vi "filter taps.vi"(8 "error in (no error)":errorcluster, 10 "filter parameters":T1={"Alpha"=0.5, "Filter Length"=6, "TX Filter"=enum."Root Raised Cos"} {"Alpha" format="%.2f"}, 11 "Samples Per Symbol (16)":i32=16) -> (2 "matched filter coefficients":dbl[](array[numeric]), 3 "pulse shaping filter coefficients":dbl[](array[numeric]) caption="Filter Coefficients" format="%.2f")   [LabVIEW 2011]
panel:
  out "Matched filter":dbl[](graph) caption="RX matched filter"
  out "Pulse shaping filter":dbl[](graph) caption="TX pulse shaping filter"
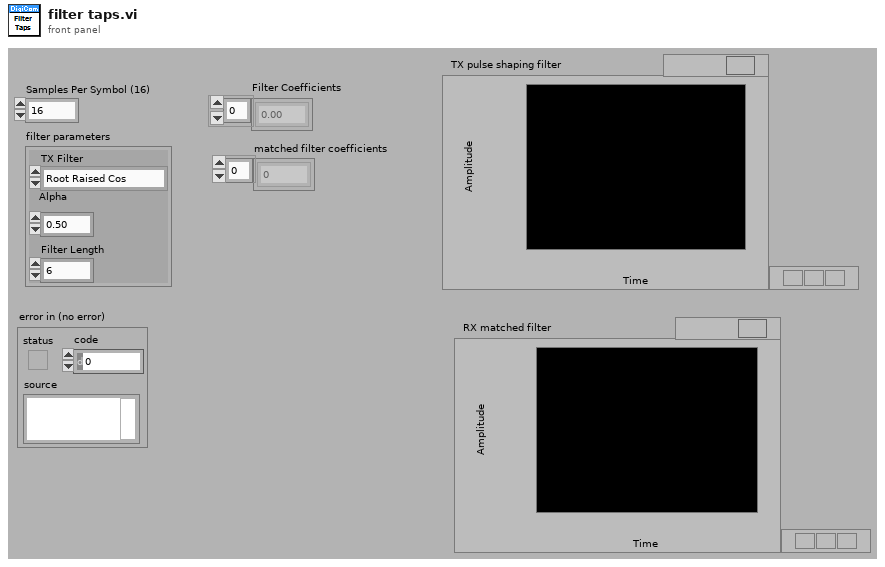
[diagram p1: front panel]
types:
  T1 = cluster{"Alpha":dbl, "Filter Length":i32, "TX Filter":enum16{"Root Raised Cos", "Raised Cos", "Rectangular"}}
  T2 = enum16{"Root Raised Cos", "Raised Cos", "Rectangular"}
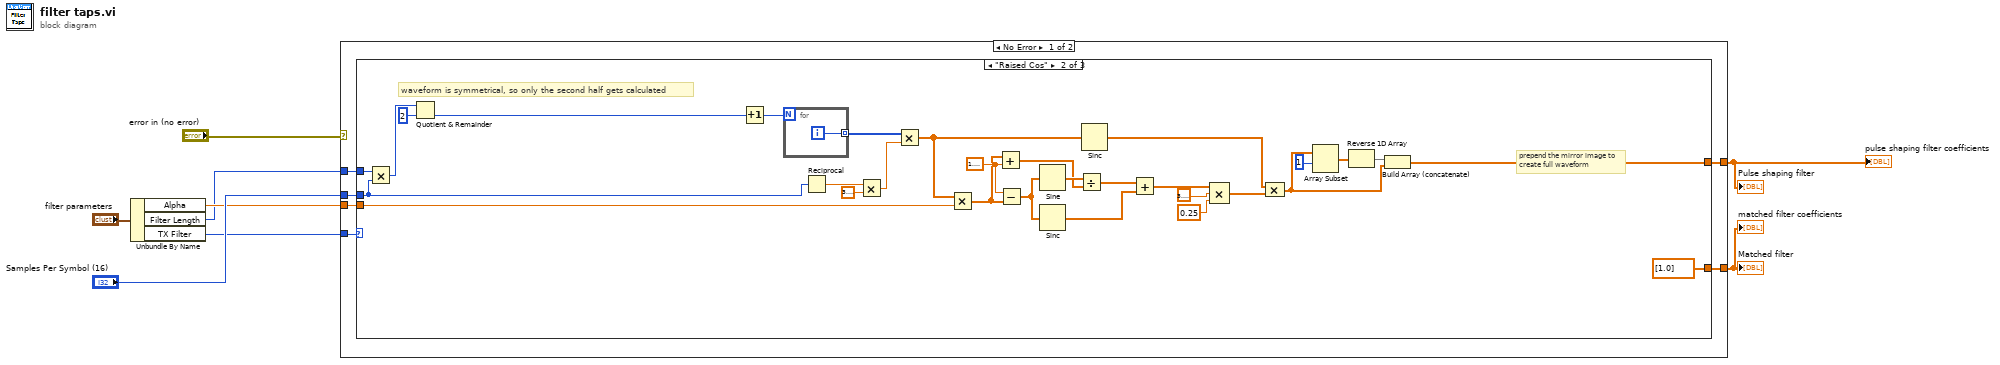
[diagram p0: block diagram]
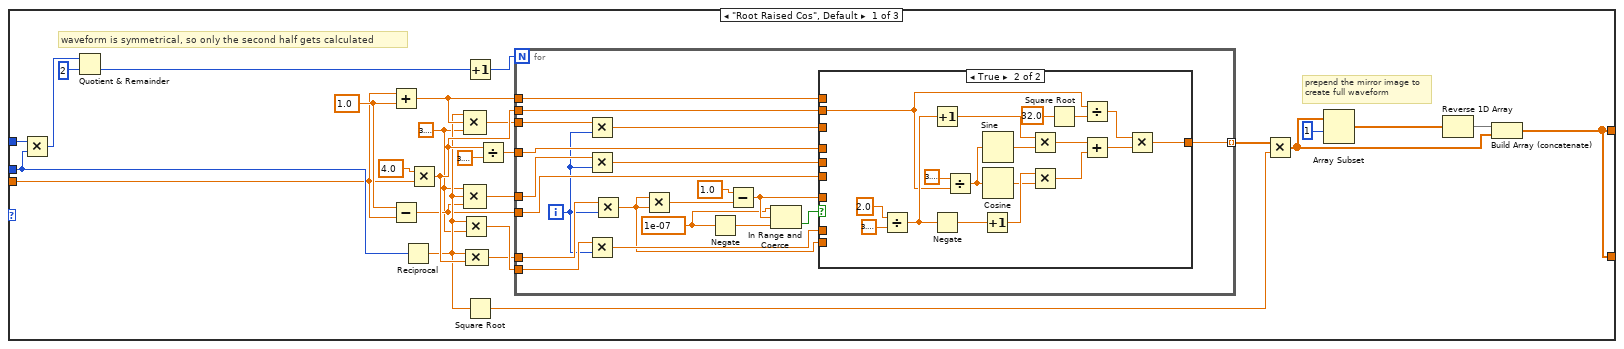
[diagram p2: hidden frame]
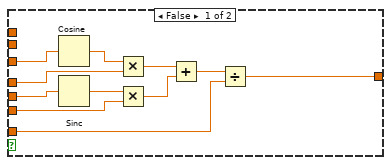
[diagram p3: hidden frame]
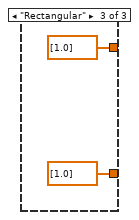
[diagram p4: hidden frame]
diagram:
  n1 = Unbundle By Name("filter parameters") -> ("Alpha"=w4:dbl, "Filter Length"=w3:i32, "TX Filter"=w2:T2)
  n2 = case shown="No Error" "error in (no error)" {
    tunnel: w3 -> [w14 _]
    tunnel: "Samples Per Symbol (16)" -> [w13 _]
    tunnel: w4 -> [w12 _]
    tunnel: [w11 _] -> w7
    tunnel: w2 -> [w10 _]
    tunnel: [w9 _] -> w1
    frame No Error {
      n3 = case shown="\"Raised Cos\"" w10 {
        tunnel: w14 -> [w17 w111 _]
        tunnel: w13 -> [w18 w110 _]
        tunnel: w12 -> [w16 w105 _]
        tunnel: [w15 w92 dbl[] [1.0] ("pulse shaping filter coefficients")] -> w11
        tunnel: [w15 dbl[] [1.0] ("matched filter coefficients") dbl[] [1.0] ("matched filter coefficients")] -> w9
        frame "Root Raised Cos", Default {
          w24 = 3.141592653589793
          w23 = 1.0 ("y")
          # "waveform is symmetrical, so only the second half gets calculated"
          # "prepend the mirror image to create full waveform"
          n4 = Multiply(x=w17, y=w18) -> (x*y=w19:i32)
          n5 = Quotient & Remainder(x=w19, y=2) -> (floor(x/y)=w22:i32)  [unwired: 1 out]
          n6 = Add(x=w16, y=w23) -> (x+y=w41:dbl)
          n7 = Subtract(x=w23, y=w16) -> (x-y=w29:dbl)
          n8 = Reciprocal(x=w18) -> (1/x=w38:dbl)
          n9 = Multiply(x=4.0 ("Input"), y=w16) -> (x*y=w40:dbl)
          n10 = Multiply(x=w38, y=w24) -> (x*y=w39:dbl)
          n11 = Compound Arithmetic op=MULTIPLY(w38, w41, w24) -> (w25:dbl)
          n12 = Compound Arithmetic op=MULTIPLY(w24, w38, w29) -> (w26:dbl)
          n13 = Increment(x=w22) -> (x+1=w21:i32)
          n14 = Square Root(x=w38) -> (sqrt(x)=w33:dbl)
          n15 = Compound Arithmetic op=MULTIPLY(w38, w40) -> (w27:dbl)
          n16 = Divide(x=w40, y=3.141592653589793) -> (x/y=w31:dbl)
          n17 = for {
            N: w21 -> [_]
            tunnel: w25 -> [w59]
            tunnel: w26 -> [w60]
            tunnel: w27 -> [w61]
            tunnel: w29 -> [w54]
            tunnel: w31 -> [w53]
            tunnel: [w52] -> w32 mode=indexing
            tunnel: w39 -> [w51]
            tunnel: w40 -> [w48]
            tunnel: w41 -> [w47]
            i -> [w50]
            w43 = 1e-07 ("y")
            n18 = Multiply(x=w59, y=w50) -> (x*y=w58:dbl)
            n19 = Multiply(x=w60, y=w50) -> (x*y=w57:dbl)
            n20 = Multiply(x=w51, y=w50) -> (x*y=w49:dbl)
            n21 = Multiply(x=w61, y=w50) -> (x*y=w46:dbl)
            n22 = Multiply(x=w46, y=w46) -> (x*y=w56:dbl)
            n23 = Negate(x=w43) -> (-x=w42:dbl)
            n24 = Subtract(x=1.0 ("y"), y=w56) -> (x-y=w44:dbl)
            n25 = In Range and Coerce(upper limit=w43, x=w44, lower limit=w42) -> (In Range?=w45:bool)  [unwired: 1 out]
            n26 = case shown="True" w45 {
              tunnel: w58 -> [w72 _]
              tunnel: w57 -> [w71 _]
              tunnel: w54 -> [w69 _]
              tunnel: w53 -> [w67 _]
              tunnel: w44 -> [w63 _]
              tunnel: [w62 w73] -> w52
              tunnel: w49 -> [_ _]
              tunnel: w48 -> [_ w78]
              tunnel: w47 -> [_ _]
              tunnel: w46 -> [_ _]
              frame False {
                n27 = Cosine(x=w72) -> (cos(x)=w68:dbl)
                n28 = Sinc(1:w71) -> (0:w70:dbl)
                n29 = Multiply(x=w68, y=w67) -> (x*y=w66:dbl)
                n30 = Multiply(x=w70, y=w69) -> (x*y=w65:dbl)
                n31 = Add(x=w66, y=w65) -> (x+y=w64:dbl)
                n32 = Divide(x=w64, y=w63) -> (x/y=w62:dbl)
              }
              frame True {
                n33 = Divide(x=2.0, y=3.141592653589793) -> (x/y=w79:dbl)
                n34 = Increment(x=w79) -> (x+1=w86:dbl)
                n35 = Negate(x=w79) -> (-x=w84:dbl)
                n36 = Divide(x=3.141592653589793, y=w78) -> (x/y=w89:dbl)
                n37 = Increment(x=w84) -> (x+1=w83:dbl)
                n38 = Sine(x=w89) -> (sin(x)=w85:dbl)
                n39 = Cosine(x=w89) -> (cos(x)=w82:dbl)
                n40 = Multiply(x=w86, y=w85) -> (x*y=w81:dbl)
                n41 = Multiply(x=w83, y=w82) -> (x*y=w80:dbl)
                n42 = Square Root(x=32.0 ("y")) -> (sqrt(x)=w76:dbl)
                n43 = Divide(x=w78, y=w76) -> (x/y=w74:dbl)
                n44 = Add(x=w81, y=w80) -> (x+y=w75:dbl)
                n45 = Multiply(x=w74, y=w75) -> (x*y=w73:dbl)
              }
            }
          }
          n46 = Multiply(x=w32, y=w33) -> (x*y=w37:dbl[])
          n47 = Array Subset(array=w37, index=1 ("Array Index")) -> (w35:dbl[])  [unwired: 1 in]
          n48 = Reverse 1D Array(array=w35) -> (reversed array=w36:dbl[])
          n49 = Build Array (concatenate)(w36, w37) -> (w15:dbl[])
        }
        frame "Raised Cos" {
          w104 = 1.5707963267948966
          # "waveform is symmetrical, so only the second half gets calculated"
          # "prepend the mirror image to create full waveform"
          n50 = Multiply(x=w111, y=w110) -> (x*y=w112:i32)
          n51 = Quotient & Remainder(x=w112, y=2) -> (floor(x/y)=w115:i32)  [unwired: 1 out]
          n52 = Increment(x=w115) -> (x+1=w114:i32)
          n53 = for {
            N: w114 -> [_]
            tunnel: [w121] -> w109 mode=indexing
            i -> [w121]
          }
          n54 = Reciprocal(x=w110) -> (1/x=w120:dbl)
          n55 = Multiply(x=w120, y=3.141592653589793) -> (x*y=w108:dbl)
          n56 = Multiply(x=w109, y=w108) -> (x*y=w106:dbl[])
          n57 = Multiply(x=w106, y=w105) -> (x*y=w103:dbl[])
          n58 = Add(x=w103, y=w104) -> (x+y=w100:dbl[])
          n59 = Subtract(x=w104, y=w103) -> (x-y=w102:dbl[])
          n60 = Sine(x=w102) -> (sin(x)=w101:dbl[])
          n61 = Sinc(1:w102) -> (0:w98:dbl[])
          n62 = Divide(x=w101, y=w100) -> (x/y=w99:dbl[])
          n63 = Sinc(1:w106) -> (0:w107:dbl[])
          n64 = Add(x=w99, y=w98) -> (x+y=w96:dbl[])
          n65 = Compound Arithmetic op=MULTIPLY(w96, 3.141592653589793, 0.25 ("value")) -> (w94:dbl[])
          n66 = Compound Arithmetic op=MULTIPLY(w107, w94) -> (w93:dbl[])
          n67 = Array Subset(array=w93, index=1 ("Array Index")) -> (w118:dbl[])  [unwired: 1 in]
          n68 = Reverse 1D Array(array=w118) -> (reversed array=w119:dbl[])
          n69 = Build Array (concatenate)(w119, w93) -> (w92:dbl[])
        }
        frame "Rectangular" {
        }
      }
    }
    frame Error {
    }
  }
  "Pulse shaping filter" <- w7
  "pulse shaping filter coefficients" <- w7
  "matched filter coefficients" <- w1
  "Matched filter" <- w1
